vi "Main.vi"(8 "error in":errorcluster, 11 "_Rename in":refnum<class "_Rename.lvclass">) -> (0 "error out":errorcluster, 3 "_Rename out":refnum<class "_Rename.lvclass">)   [LabVIEW 2020, in "_Rename.lvlib" / "_Rename.lvclass"]
uses:
  _Rename.lvclass
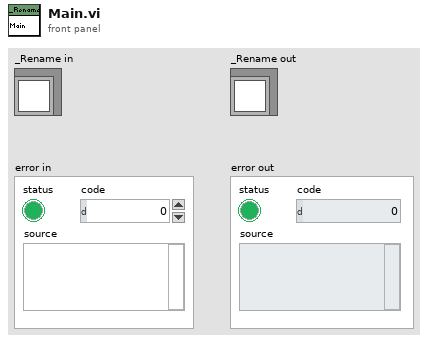
[diagram p1: front panel]
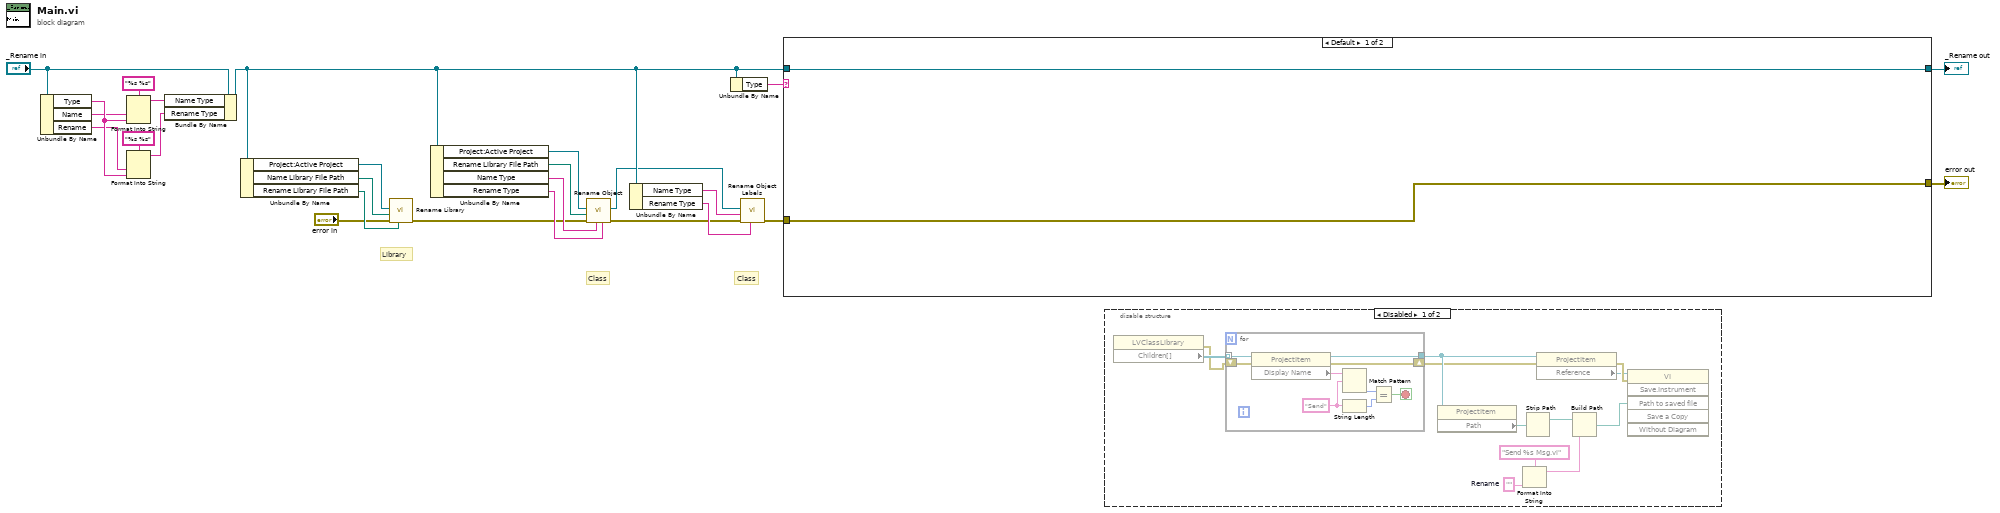
[diagram p0: block diagram]
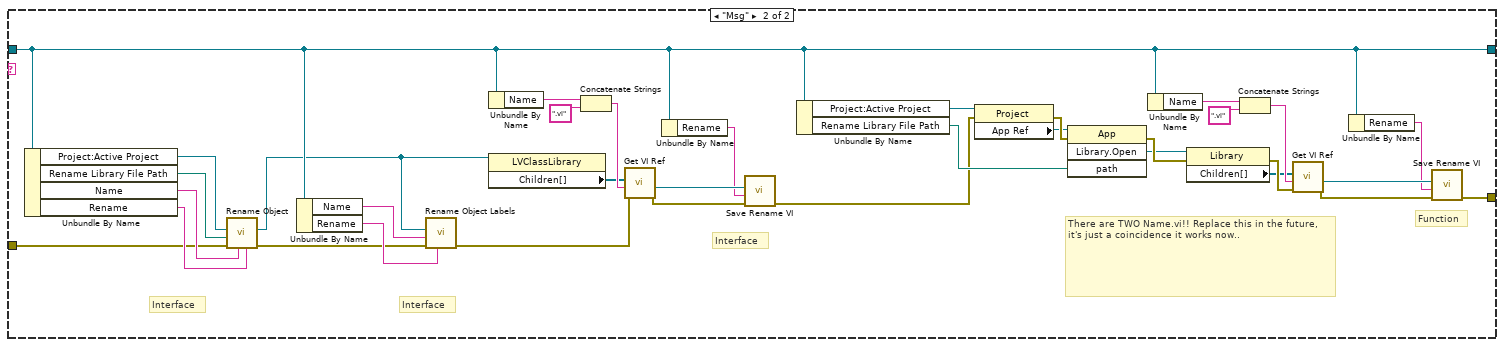
[diagram p3: hidden frame]
diagram:
  # "Class"
  # "Library"
  # "Class"
  n1 = Unbundle By Name("_Rename in") -> ("Type"=w22:string, "Name"=w20:string, "Rename"=w21:string)
  n2 = Format Into String(format string="%s %s", w20, w22) -> (resulting string=w19:string)  [unwired: 2 in, 1 out]
  n3 = Format Into String(format string="%s %s", w21, w22) -> (resulting string=w18:string)  [unwired: 2 in, 1 out]
  n4 = Bundle By Name(cluster="_Rename in", "Name Type"=w19, "Rename Type"=w18) -> (w6:refnum<class "_Rename.lvclass">)
  n5 = Unbundle By Name(w6) -> ("Project:Active Project"=w8:refnum<vi>, "Name Library File Path"=w10:path, "Rename Library File Path"=w9:path)
  n6 = call "Rename Library.vi"("Rename Library File Path"=w9, "error in"="error in", "Name Library File Path"=w10, "Project:Active Project"=w8) -> ("error out"=w11:errorcluster)  [unwired: 7 in]
  n7 = Unbundle By Name(w6) -> ("Project:Active Project"=w12:refnum<vi>, "Rename Library File Path"=w13:path, "Name Type"=w14:string, "Rename Type"=w15:string)
  n8 = call "Rename Object.vi"("Post"=w15, "Pre"=w14, "error in"=w11, "Rename Library File Path"=w13, "Project:Active Project"=w12) -> ("error out"=w16:errorcluster, "Object Ref"=w5:refnum<vi>)  [unwired: 5 in]
  n9 = Unbundle By Name(w6) -> ("Name Type"=w26:string, "Rename Type"=w25:string)
  n10 = Unbundle By Name(w6) -> ("Type"=w7:string)
  n11 = call "Rename Object Labels.vi"("Post"=w25, "error in"=w16, "Pre"=w26, "Class Ref"=w5) -> ("error out"=w4:errorcluster)  [unwired: 7 in]
  n12 = case shown="Default" w7 {
    tunnel: w4 -> [w28 w29]
    tunnel: [w28 w33] -> w2
    tunnel: [w27 w47] -> w3
    tunnel: w6 -> [w27 w47]
    frame Default {
    }
    frame "Msg" {
      # "There are TWO Name.vi!! Replace this in the future, it's just a coincidence it works now.."
      # "Interface"
      # "Function"
      # "Interface"
      # "Interface"
      n13 = Unbundle By Name(w47) -> ("Project:Active Project"=w56:refnum<vi>, "Rename Library File Path"=w57:path, "Name"=w58:string, "Rename"=w59:string)
      n14 = call "Rename Object.vi"("Post"=w59, "Pre"=w58, "error in"=w29, "Rename Library File Path"=w57, "Project:Active Project"=w56) -> ("error out"=w60:errorcluster, "Object Ref"=w42:refnum<vi>)  [unwired: 5 in]
      n15 = Unbundle By Name(w47) -> ("Name"=w62:string, "Rename"=w61:string)
      n16 = call "Rename Object Labels.vi"("Post"=w61, "error in"=w60, "Pre"=w62, "Class Ref"=w42) -> ("error out"=w52:errorcluster)  [unwired: 7 in]
      n17 = Unbundle By Name(w47) -> ("Name"=w55:string)
      n18 = property class="LVClassLibrary"(reference=w42) -> ("Children[]"=w41:refnum<vi>[])  [unwired: 1 in, 2 out]
      n19 = Concatenate Strings(w55, ".vi" ("string")) -> (w53:string)
      n20 = call "Get VI Ref.vi"("error in"=w52, "Name.vi"=w53, "Owned Items[]"=w41) -> ("error out"=w35:errorcluster, "VI Reference"=w37:refnum<vi>)  [unwired: 7 in]
      n21 = Unbundle By Name(w47) -> ("Rename"=w36:string)
      n22 = call "Save Rename VI.vi"("error in"=w35, "Rename"=w36, "VI Ref"=w37) -> ("error out"=w34:errorcluster)  [unwired: 8 in]
      n23 = Unbundle By Name(w47) -> ("Project:Active Project"=w46:refnum<vi>, "Rename Library File Path"=w45:path)
      n24 = property class="Project"(reference=w46, error in=w34) -> (error out=w49:errorcluster, "App Ref"=w48:refnum<vi>)  [unwired: 1 out]
      n25 = invoke class="App" method="Library.Open"(reference=w48, error in=w49, "path"=w45) -> (error out=w44:errorcluster, "Open Library"=w43:refnum<vi>)  [unwired: 1 in, 2 out]
      n26 = Unbundle By Name(w47) -> ("Name"=w51:string)
      n27 = property class="Library"(reference=w43, error in=w44) -> (error out=w39:errorcluster, "Children[]"=w38:refnum<vi>[])  [unwired: 1 out]
      n28 = Concatenate Strings(w51, ".vi" ("string")) -> (w40:string)
      n29 = call "Get VI Ref.vi"("error in"=w39, "Name.vi"=w40, "Owned Items[]"=w38) -> ("error out"=w32:errorcluster, "VI Reference"=w31:refnum<vi>)  [unwired: 7 in]
      n30 = Unbundle By Name(w47) -> ("Rename"=w30:string)
      n31 = call "Save Rename VI.vi"("error in"=w32, "Rename"=w30, "VI Ref"=w31) -> ("error out"=w33:errorcluster)  [unwired: 8 in]
    }
  }
  "_Rename out" <- w3
  "error out" <- w2
  n32 = disable-structure shown="Disabled" {
    frame Disabled {
      w67 = ""  # Rename
      n33 = property class="LVClassLibrary"() -> (error out=w65:errorcluster, "Children[]"=w66:refnum<vi>[])  [unwired: 2 in, 1 out]
      n34 = for {
        tunnel: w66 -> [w83] mode=indexing
        shift-right: [w81] -> w63
        shift-left: w65 -> [w82]
        tunnel: [w80] -> w64
        stop <- w78 stop-if-true
        w75 = "Send" ("string")
        n35 = property class="ProjectItem"(reference=w83, error in=w82) -> (reference out=w80:refnum<vi>, error out=w81:errorcluster, "Display Name"=w79:string)
        n36 = Match Pattern(string=w79, regular expression=w75) -> (offset past match=w77:i32)  [unwired: 1 in, 3 out]
        n37 = String Length(string=w75) -> (length=w76:i32)
        n38 = Equal?(x=w77, y=w76) -> (x = y?=w78:bool)
      }
      n39 = property class="ProjectItem"(reference=w64) -> ("Path"=w70:path)  [unwired: 1 in, 2 out]
      n40 = Format Into String(format string="Send %s Msg.vi", w67) -> (resulting string=w68:string)  [unwired: 2 in, 1 out]
      n41 = Strip Path(path=w70) -> (stripped path=w73:path)  [unwired: 1 out]
      n42 = property class="ProjectItem"(reference=w64, error in=w63) -> (error out=w74:errorcluster, "Reference"=w72:refnum<vi>)  [unwired: 1 out]
      n43 = Build Path(base path=w73, name or relative path=w68) -> (appended path=w71:path)
      n44 = invoke class="VI" method="Save.Instrument"(reference=w72, error in=w74, "Path to saved file"=w71) -> ()  [unwired: 3 in, 6 out]
    }
    frame Enabled {
    }
  }
